vi "S2C_FPGA_I16ToDouble.vi"(4 "I16 In":i16 format="%x") -> (1 "Double Out":dbl min=-10.0 max=10.0 step=0.0003000000142492354 format="%#.6g")   [LabVIEW 2015]
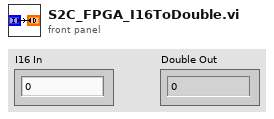
[diagram p1: front panel]
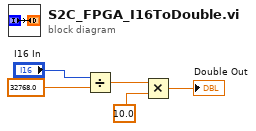
[diagram p0: block diagram]
diagram:
  n1 = Divide(x="I16 In", y=32768.0) -> (x/y=w4:dbl)
  n2 = Multiply(x=w4, y=10.0) -> (x*y=→"Double Out":dbl)
